vi "getTemperatureTarget.vi"(6 "Channel":i32, 8 "error in (no error)":errorcluster, 11 "Instrument.Cryostat in":refnum<class "Instrument.Cryostat.lvclass">) -> (0 "error out":errorcluster, 1 "Status":string, 2 "Temperature (K)":dbl, 3 "Instrument.Cryostat out":refnum<class "Instrument.Cryostat.lvclass">, 4 "Finished?":bool)   [LabVIEW 2019, in "Instrument.Cryostat.lvclass"]
uses:
  Instrument.Cryostat.lvclass
  Typedefs/getTemperature--cluster.ctl
  Typedefs/Cryostat.commands--enum.ctl
  41387025-2c78-49fb-8ab2-79a0639f242c.vi
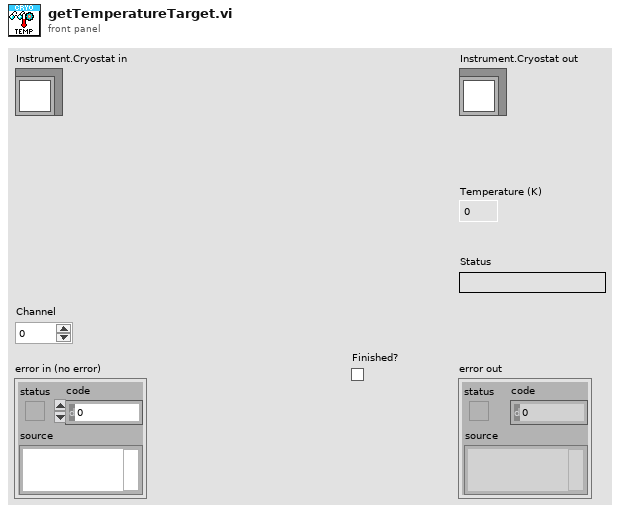
[diagram p1: front panel]
types:
  T1 = typedef "Instrument.Cryostat.lvclass/Cryostat.commands--enum.ctl" = enum16{"getLN2Level", "getLHeLevel", "getMagnet", "getMagnetVector", "getMagnetTarget", "getMagnetVectorTarget", "setMagnet", "setMagnetVector", "getAngle", "setAngle", "getTemperature", "getTemperatureTarget", "setTemperature", "getHeater", "setHeater", "getChamber", "setChamber", "getPressure"}
  T2 = typedef "Instrument.Cryostat.lvclass/getTemperature--cluster.ctl" = cluster{"temperature":dbl, "status":string, "finished":bool}
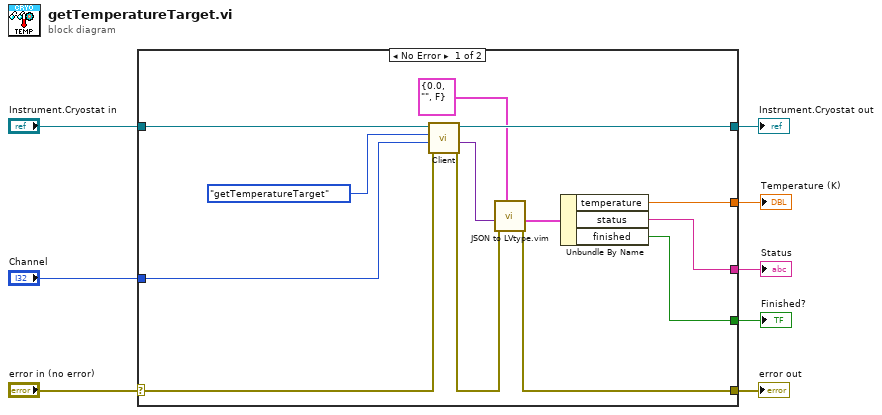
[diagram p0: block diagram]
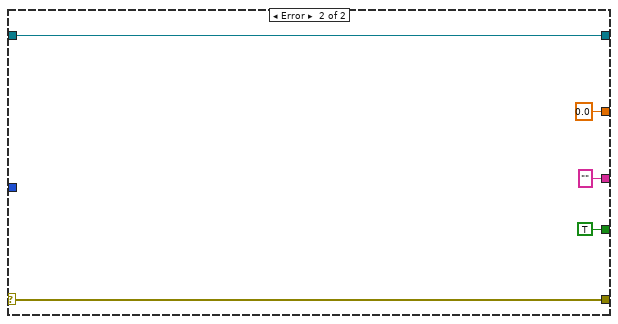
[diagram p2: hidden frame]
diagram:
  n1 = case shown="No Error" "error in (no error)" {
    selector: "error in (no error)" -> [w14 w26]
    tunnel: [w9 w26] -> w7
    tunnel: [w21 w25] -> w5
    tunnel: "Instrument.Cryostat in" -> [w15 w25]
    tunnel: [w20 0.0 ("Temperature (K)")] -> w4
    tunnel: [w19 "" ("Status")] -> w3
    tunnel: [w18 TRUE ("Finished?")] -> w2
    tunnel: "Channel" -> [w17 _]
    frame No Error {
      n2 = call-dynamic "Client.vi"("error in (no error)"=w14, "Data in"=w17, "Command in"=Cryostat.commands--enum."getTemperatureTarget" ("commands"), "Instrument in"=w15) -> ("error out"=w11:errorcluster, "Data out"=w12:variant, "Instrument out"=w21:refnum<class "Instrument.Cryostat.lvclass">)  [unwired: 4 in, 1 out]
      n3 = call "JSON to LVtype.vim"("type"=T2 {"temperature"=0.0, "status"="", "finished"=FALSE} ("getTemperature"), "error in (no error)"=w11, "JSON Data in"=w12) -> ("error out"=w9:errorcluster, "Data out"=w10:T2)  [unwired: 7 in]
      n4 = Unbundle By Name(w10) -> ("temperature"=w20:dbl, "status"=w19:string, "finished"=w18:bool)
    }
    frame Error {
    }
  }
  "error out" <- w7
  "Instrument.Cryostat out" <- w5
  "Temperature (K)" <- w4
  "Status" <- w3
  "Finished?" <- w2
